vi "Update parameters (array).vi"(10 "New Parameters":cluster{"Name":string, "Value":string}[](array[cluster]), 11 "Parameters":cluster{"Name":string, "Value":string}[](array[cluster])) -> (3 "Parameters Out":cluster{"Name":string, "Value":string}[](array[cluster]))   [LabVIEW 2020, in "Measurement.lvclass"]
uses:
  Measurement.lvclass
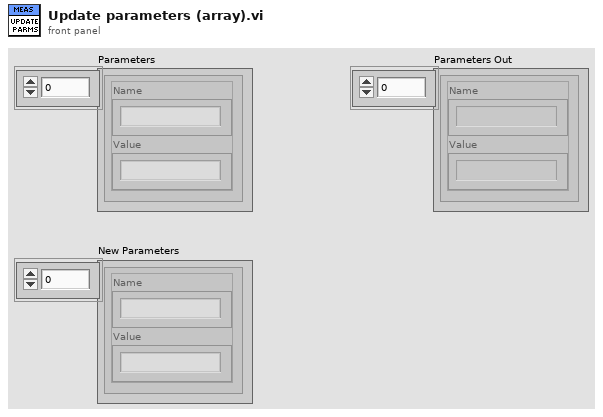
[diagram p1: front panel]
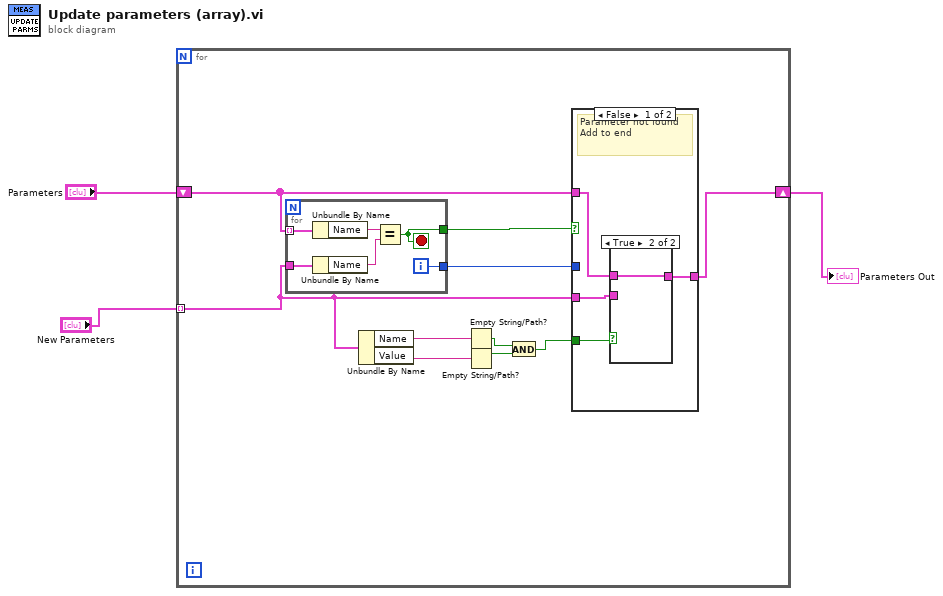
[diagram p0: block diagram]
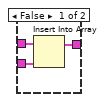
[diagram p2: hidden frame]
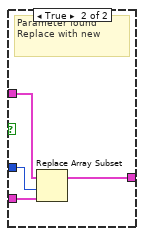
[diagram p3: hidden frame]
diagram:
  n1 = for {
    shift-right: [w10] -> w2
    shift-left: "Parameters" -> [w11]
    tunnel: "New Parameters" -> [w4] mode=indexing
    n2 = for {
      tunnel: w11 -> [w31] mode=indexing
      tunnel: w4 -> [w30]
      tunnel: [w27] -> w13
      tunnel: [w26] -> w12
      i -> [w26]
      stop <- w27 stop-if-true
      n3 = Unbundle By Name(w31) -> ("Name"=w29:string)
      n4 = Unbundle By Name(w30) -> ("Name"=w28:string)
      n5 = Equal?(x=w29, y=w28) -> (x = y?=w27:bool)
    }
    n6 = Unbundle By Name(w4) -> ("Name"=w9:string, "Value"=w8:string)
    n7 = Empty String/Path?(string/path=w9) -> (empty?=w7:bool)
    n8 = Empty String/Path?(string/path=w8) -> (empty?=w6:bool)
    n9 = And(x=w7, y=w6) -> (x .and. y?=w5:bool)
    n10 = case shown="False" w13 {
      tunnel: w12 -> [_ w24]
      tunnel: w11 -> [w17 w25]
      tunnel: w4 -> [w15 w23]
      tunnel: [w16 w22] -> w10
      tunnel: w5 -> [w14 _]
      frame False {
        # "Parameter not found\nAdd to end"
        n11 = case shown="True" w14 {
          tunnel: w17 -> [w20 w21]
          tunnel: [w19 w21] -> w16
          tunnel: w15 -> [w18 _]
          frame False {
            n12 = Insert Into Array(array=w20, new element=w18) -> (w19:cluster{"Name":string, "Value":string}[])  [unwired: 1 in]
          }
          frame True {
          }
        }
      }
      frame True {
        # "Parameter found\nReplace with new"
        n13 = Replace Array Subset(array=w25, new element=w23, index=w24) -> (w22:cluster{"Name":string, "Value":string}[])
      }
    }
  }
  "Parameters Out" <- w2
